vi "Wizard Array Enqueue Function.vi"(0 "Qref in":refnum<queue>, 7 "Array of Messages":T1[](array[typedef])=[{"State"=enum."Initialize 0", "Data"=variant}], 11 "Error in":errorcluster, 13 "Mode":enum16{"Back", "Front", "Replace"}(ring)) -> (4 "Qref out":refnum<queue>, 15 "Error out":errorcluster)   [LabVIEW 2014]
uses:
  TypeDef and Controls/QWizardMessage.ctl
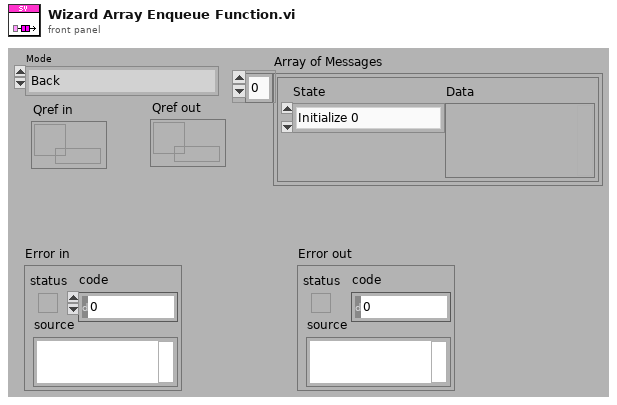
[diagram p1: front panel]
types:
  T1 = typedef "QWizardMessage.ctl" = cluster{"State":enum16{"Initialize 0", "Initialize 1", "Initialize 2", "Initialize 3", "Initialize 4", "Back", "Next", "Check Database", "Get Lib Name", "Get Lib Folder", "Get Database", "Check Lib Availability", "Create SV Lib", "Check Binding", "Bind", "Get Processes", "Deploy", "Remove Process", "Clear Engine", "Initialize Process", "Get Process AP2", "Update Var AP2", "Import", "Redo", "Save Database", "Exit"}, "Data":variant}
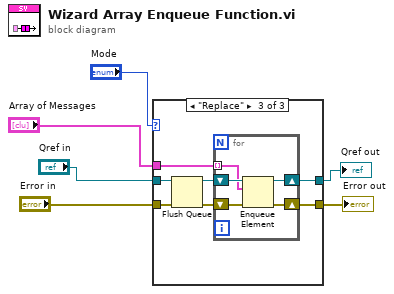
[diagram p0: block diagram]
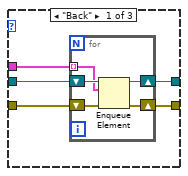
[diagram p2: hidden frame]
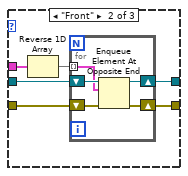
[diagram p3: hidden frame]
diagram:
  n1 = case shown="\"Replace\"" "Mode" {
    tunnel: "Array of Messages" -> [w9 w22 w32]
    tunnel: "Qref in" -> [w11 w20 w34]
    tunnel: [w10 w19 w31] -> w2
    tunnel: "Error in" -> [w8 w18 w29]
    tunnel: [w7 w17 w28] -> w6
    frame "Back" {
      n2 = for {
        shift-right: [w15] -> w10
        shift-left: w11 -> [w16]
        tunnel: w9 -> [w14] mode=indexing
        shift-right: [w12] -> w7
        shift-left: w8 -> [w13]
        n3 = Enqueue Element(queue=w16, element=w14, error in (no error)=w13) -> (queue out=w15:refnum<queue>, error out=w12:errorcluster)  [unwired: 1 in, 1 out]
      }
    }
    frame "Front" {
      n4 = Reverse 1D Array(array=w22) -> (reversed array=w21:T1[])
      n5 = for {
        tunnel: w21 -> [w26] mode=indexing
        shift-right: [w25] -> w19
        shift-left: w20 -> [w27]
        shift-right: [w23] -> w17
        shift-left: w18 -> [w24]
        n6 = Enqueue Element At Opposite End(queue=w27, element=w26, error in (no error)=w24) -> (queue out=w25:refnum<queue>, error out=w23:errorcluster)  [unwired: 1 in, 1 out]
      }
    }
    frame "Replace" {
      n7 = Flush Queue(queue=w34, error in (no error)=w29) -> (queue out=w33:refnum<queue>, error out=w30:errorcluster)  [unwired: 1 out]
      n8 = for {
        tunnel: w32 -> [w38] mode=indexing
        shift-right: [w37] -> w31
        shift-left: w33 -> [w39]
        shift-right: [w35] -> w28
        shift-left: w30 -> [w36]
        n9 = Enqueue Element(queue=w39, element=w38, error in (no error)=w36) -> (queue out=w37:refnum<queue>, error out=w35:errorcluster)  [unwired: 1 in, 1 out]
      }
    }
  }
  "Error out" <- w6
  "Qref out" <- w2
